vi "AutoSequencer.vi"(2 "Reinit Sequencer":bool, 7 "Auto Cluster In":T1) -> (8 "Auto Cluster Out":T1)   [LabVIEW 2020]
doc: "This VI manages the autonomous sequence. The drive base and manipulator sequencers operate in parallel. Autonomous plays are written as text files and uploaded to the roboRIO via FileZilla. The appropriate play is slected prior to the match via the FRC 4265 Dashboard. For each sequencer, each step is composed of a command and a parameter string of arbitrary length. The drive sequencer selects commands using a case structure while the subsystem sequencer selects commands using static VI references (this disparate choice is made due to conflicting memory handling and ease-of-creation tradeoffs). Error checking and handling is supported. An autonomous test mode (for simulating autonomous plays on the robot cart) is supported. Status updates are sent to the FRC Driver Station and the FRC 4265 Dashboard throughout autonomous. Note that the autonomous sequencer may be also active during the begining of TeleOperated mode, as determined by the MasterRobotModeController.vi."
uses:
  a18db1b9-ed6f-48db-83ed-89b9a31e5ef5.vi
  3b074430-bbfe-494f-99f2-72c3d74da684.vi
  a18db1b9-ed6f-48db-83ed-89b9a31e5ef5.vi/77c742ae-e671-49bb-a825-a6e8cebc9f63.vi
  3b074430-bbfe-494f-99f2-72c3d74da684.vi/77c742ae-e671-49bb-a825-a6e8cebc9f63.vi
  sensordata.vi
  driverdata.vi
  robotconstants.vi
  autonomousinfo.vi
  <vilib>/Rock Robotics/Network Tables/NT Write Value.vi
  <vilib>/Rock Robotics/Network Tables/NT Write String.vi
panel:
  in  "Type Def":T1
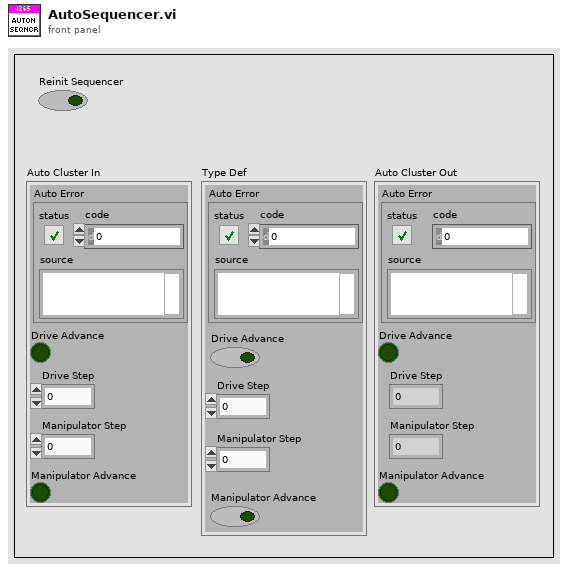
[diagram p1: front panel]
types:
  T1 = cluster{"Auto Error":errorcluster, "Drive Advance":bool, "Drive Step":i32, "Manipulator Step":i32, "Manipulator Advance":bool}
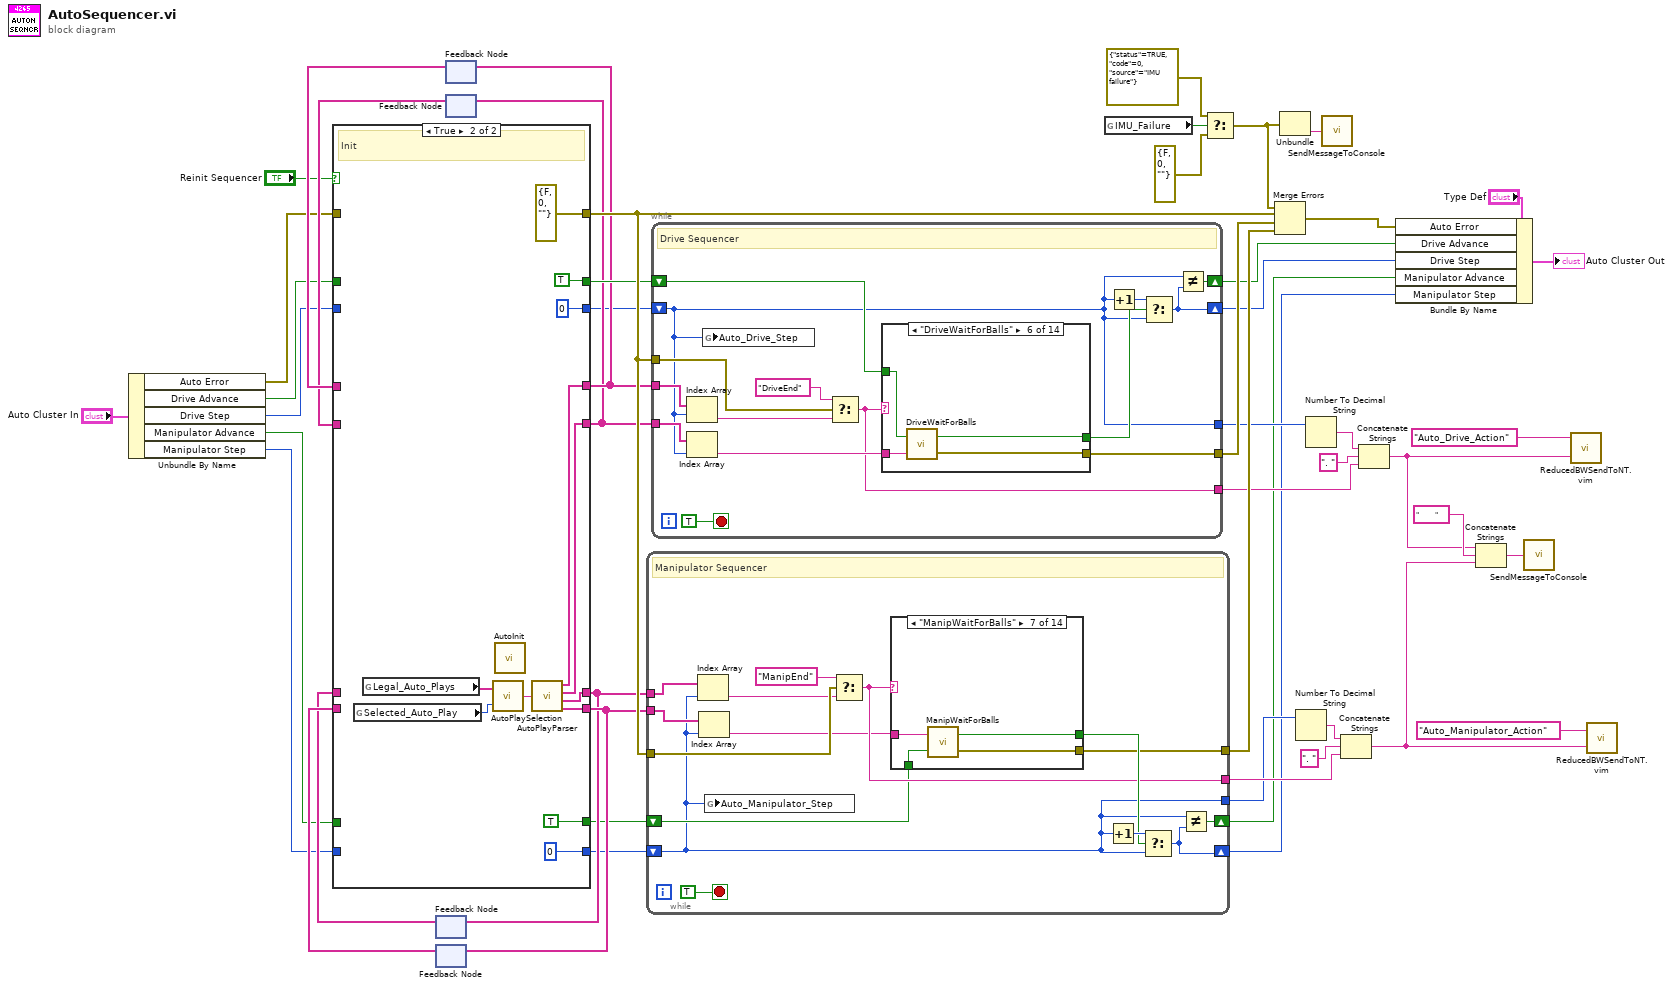
[diagram p0: block diagram]
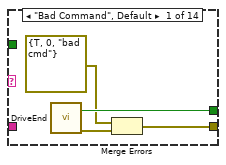
[diagram p2: hidden frame]
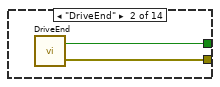
[diagram p3: hidden frame]
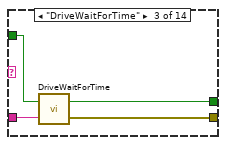
[diagram p4: hidden frame]
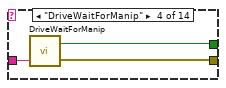
[diagram p5: hidden frame]
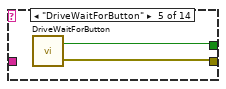
[diagram p6: hidden frame]
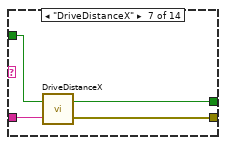
[diagram p7: hidden frame]
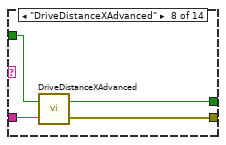
[diagram p8: hidden frame]
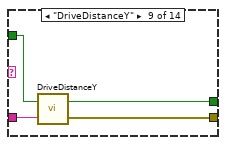
[diagram p9: hidden frame]
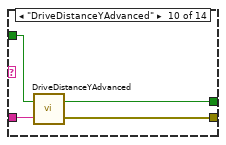
[diagram p10: hidden frame]
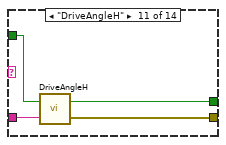
[diagram p11: hidden frame]
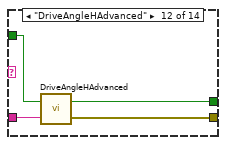
[diagram p12: hidden frame]
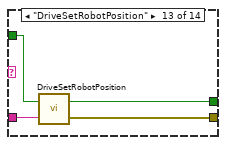
[diagram p13: hidden frame]
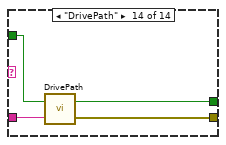
[diagram p14: hidden frame]
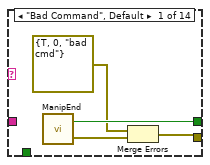
[diagram p16: hidden frame]
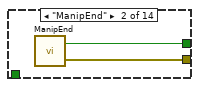
[diagram p17: hidden frame]
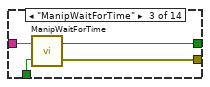
[diagram p18: hidden frame]
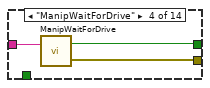
[diagram p19: hidden frame]
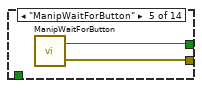
[diagram p20: hidden frame]
diagram:
  n1 = Unbundle By Name("Auto Cluster In") -> ("Auto Error"=w5:errorcluster, "Drive Advance"=w4:bool, "Drive Step"=w3:i32, "Manipulator Advance"=w2:bool, "Manipulator Step"=w1:i32)
  n2 = feedback #1() -> (w38:string[])  [unwired: 1 in]
  n3 = feedback #2() -> (w39:string[])  [unwired: 1 in]
  n4 = feedback #3() -> (w44:string[])  [unwired: 1 in]
  n5 = feedback #4() -> (w43:string[])  [unwired: 1 in]
  n6 = case shown="True" "Reinit Sequencer" {
    tunnel: w1 -> [w56 _]
    tunnel: w2 -> [w57 _]
    tunnel: [w57 TRUE ("Advance Trigger")] -> w25
    tunnel: [w56 0] -> w34
    tunnel: [w55 w63] -> w36
    tunnel: [w54 w67] -> w37
    tunnel: w38 -> [w55 _]
    tunnel: w39 -> [w54 _]
    tunnel: [w53 0] -> w40
    tunnel: w3 -> [w53 _]
    tunnel: [w52 w65] -> w41
    tunnel: [w51 w64] -> w42
    tunnel: w43 -> [w52 _]
    tunnel: w44 -> [w51 _]
    tunnel: [w50 TRUE] -> w45
    tunnel: w4 -> [w50 _]
    tunnel: [w49 errorcluster {"status"=FALSE, "code"=0, "source"=""} ("error constant")] -> w47
    tunnel: w5 -> [w49 _]
    frame False {
      # "Pass"
    }
    frame True {
      # "Init"
      n7 = global read "driverdata.vi" "Selected_Auto_Play"() -> (w61:u16)
      n8 = global read "robotconstants.vi" "Legal_Auto_Plays"() -> (w58:string[])
      n9 = call "AutoPlaySelection.vi"("Selected Auto Play"=w61, "Auto Plays"=w58) -> ("Autonomous Commands"=w60:string)
      n10 = call "AutoInit.vi"() -> ()  [unwired: 1 in]
      n11 = call "AutoPlayParser.vi"("Auto Play"=w60) -> ("Drive Command Strings"=w64:string[], "Drive Parameter Strings"=w65:string[], "Manipulator Command Strings"=w63:string[], "Manipulator Parameter Strings"=w67:string[])
    }
  }
  n12 = feedback-in #1(w36) -> ()
  n13 = feedback-in #2(w37) -> ()
  n14 = feedback-in #3(w42) -> ()
  n15 = feedback-in #4(w41) -> ()
  n16 = while {
    tunnel: w36 -> [w80]
    shift-right: [w82] -> w9
    shift-left: w34 -> [w70]
    shift-right: [w81] -> w10
    shift-left: w25 -> [w72]
    tunnel: w37 -> [w79]
    tunnel: [w74] -> w28
    tunnel: [w75] -> w48
    tunnel: w47 -> [w77]
    tunnel: [w70] -> w17
    stop <- TRUE stop-if-true
    # "Manipulator Sequencer"
    n17 = Index Array(array=w80, index=w70) -> (element=w71:string)
    n18 = Index Array(array=w79, index=w70) -> (element=w73:string)
    n19 = global write "autonomousinfo.vi" "Auto_Manipulator_Step"(w70) -> ()
    n20 = Select(t="ManipEnd", s=w77, f=w71) -> (s? t:f=w74:string)
    n21 = case shown="\"ManipWaitForBalls\"" w74 {
      tunnel: w73 -> [_ _ w94 w97 _ w103 w107 w110 w113 w116 w119 w122 w125 w128]
      tunnel: [w88 w90 w92 w96 w99 w101 w104 w109 w112 w115 w118 w121 w124 w127] -> w76
      tunnel: [w86 w89 w91 w95 w98 w100 w105 w108 w111 w114 w117 w120 w123 w126] -> w75
      tunnel: w72 -> [_ _ w93 _ _ w102 w106 _ _ _ _ _ _ _]
      frame "Bad Command", Default {
        n22 = call "ManipEnd.vi"() -> ("Error Out"=w87:errorcluster, "Advance Trigger"=w88:bool)  [unwired: 2 in]
        n23 = Merge Errors(errorcluster {"status"=TRUE, "code"=0, "source"="bad cmd"} ("Path Follow Error"), w87) -> (w86:errorcluster)
      }
      frame "ManipEnd" {
        n24 = call "ManipEnd.vi"() -> ("Error Out"=w89:errorcluster, "Advance Trigger"=w90:bool)  [unwired: 2 in]
      }
      frame "ManipWaitForTime" {
        n25 = call "ManipWaitForTime.vi"("Reinit"=w93, "Parameter String"=w94) -> ("Error Out"=w91:errorcluster, "Increment"=w92:bool)
      }
      frame "ManipWaitForDrive" {
        n26 = call "ManipWaitForDrive.vi"("Parameter String"=w97) -> ("Error Out"=w95:errorcluster, "Increment"=w96:bool)  [unwired: 1 in]
      }
      frame "ManipWaitForButton" {
        n27 = call "ManipWaitForButton.vi"() -> ("Error Out"=w98:errorcluster, "Increment"=w99:bool)  [unwired: 2 in]
      }
      frame "ManipWaitForDistance" {
        n28 = call "ManipWaitForDistance.vi"("Reinit"=w102, "Parameter String"=w103) -> ("Error Out"=w100:errorcluster, "Increment"=w101:bool)
      }
      frame "ManipWaitForBalls" {
        n29 = call "ManipWaitForBalls.vi"("Reinit"=w106, "Parameter String"=w107) -> ("Error Out"=w105:errorcluster, "Increment"=w104:bool)
      }
      frame "ManipIntake" {
        n30 = call "ManipIntake.vi"("Instruction String"=w110) -> ("Error Out"=w108:errorcluster, "Advance Trigger"=w109:bool)  [unwired: 1 in]
      }
      frame "ManipShootBalls" {
        n31 = call "ManipShootBalls.vi"("Instruction String"=w113) -> ("Error Out"=w111:errorcluster, "Advance Trigger"=w112:bool)  [unwired: 1 in]
      }
      frame "ManipForceFire" {
        n32 = call "ManipForceFire.vi"("Instruction String"=w116) -> ("Error Out"=w114:errorcluster, "Advance Trigger"=w115:bool)  [unwired: 1 in]
      }
      frame "ManipChangeState" {
        n33 = call "ManipChangeState.vi"("Instruction String"=w119) -> ("Error Out"=w117:errorcluster, "Advance Trigger"=w118:bool)  [unwired: 1 in]
      }
      frame "ManipPrespin" {
        n34 = call "ManipPrespin.vi"("Instruction String"=w122) -> ("Error Out"=w120:errorcluster, "Advance Trigger"=w121:bool)  [unwired: 1 in]
      }
      frame "ManipSetPreloadBalls" {
        n35 = call "ManipSetPreloadBalls.vi"("Parameter String"=w125) -> ("Error Out"=w123:errorcluster, "Increment"=w124:bool)  [unwired: 9 in]
      }
      frame "ManipHumanPlayerSignal" {
        n36 = call "ManipHumanPlayerSignal.vi"("Instruction String"=w128) -> ("Error Out"=w126:errorcluster, "Advance Trigger"=w127:bool)  [unwired: 9 in]
      }
    }
    n37 = Increment(x=w70) -> (x+1=w84:i32)
    n38 = Select(t=w84, s=w76, f=w70) -> (s? t:f=w82:i32)
    n39 = Not Equal?(x=w70, y=w82) -> (x != y?=w81:bool)
  }
  n40 = while {
    shift-right: [w138] -> w11
    shift-left: w40 -> [w129]
    tunnel: w42 -> [w141]
    tunnel: w41 -> [w140]
    shift-right: [w137] -> w12
    shift-left: w45 -> [w136]
    tunnel: [w130] -> w33
    tunnel: w47 -> [w134]
    tunnel: [w131] -> w46
    tunnel: [w129] -> w18
    stop <- TRUE stop-if-true
    # "Drive Sequencer"
    n41 = Index Array(array=w141, index=w129) -> (element=w133:string)
    n42 = Index Array(array=w140, index=w129) -> (element=w139:string)
    n43 = global write "autonomousinfo.vi" "Auto_Drive_Step"(w129) -> ()
    n44 = Select(t="DriveEnd", s=w134, f=w133) -> (s? t:f=w130:string)
    n45 = case shown="\"DriveWaitForBalls\"" w130 {
      tunnel: w139 -> [_ _ w151 w156 _ w162 w165 w169 w172 w177 w180 w185 w189 w193]
      tunnel: [w147 w149 w152 w154 w158 w160 w164 w168 w174 w176 w182 w184 w190 w191] -> w135
      tunnel: w136 -> [_ _ w150 _ _ w159 w166 w170 w173 w178 w181 w186 w188 w194]
      tunnel: [w145 w148 w153 w155 w157 w161 w163 w167 w171 w175 w179 w183 w187 w192] -> w131
      frame "Bad Command", Default {
        n46 = call "DriveEnd.vi"() -> ("Error Out"=w146:errorcluster, "Advance Trigger"=w147:bool)  [unwired: 2 in]
        n47 = Merge Errors(errorcluster {"status"=TRUE, "code"=0, "source"="bad cmd"} ("Path Follow Error"), w146) -> (w145:errorcluster)
      }
      frame "DriveEnd" {
        n48 = call "DriveEnd.vi"() -> ("Error Out"=w148:errorcluster, "Advance Trigger"=w149:bool)  [unwired: 2 in]
      }
      frame "DriveWaitForTime" {
        n49 = call "DriveWaitForTime.vi"("Parameter String"=w151, "Reinit"=w150) -> ("Error Out"=w153:errorcluster, "Increment"=w152:bool)
      }
      frame "DriveWaitForManip" {
        n50 = call "DriveWaitForManip.vi"("Parameter String"=w156) -> ("Error Out"=w155:errorcluster, "Increment"=w154:bool)  [unwired: 1 in]
      }
      frame "DriveWaitForButton" {
        n51 = call "DriveWaitForButton.vi"() -> ("Error Out"=w157:errorcluster, "Increment"=w158:bool)  [unwired: 2 in]
      }
      frame "DriveWaitForBalls" {
        n52 = call "DriveWaitForBalls.vi"("Parameter String"=w162, "Reinit"=w159) -> ("Error Out"=w161:errorcluster, "Increment"=w160:bool)
      }
      frame "DriveDistanceX" {
        n53 = call "DriveDistanceX.vi"("Parameter String"=w165, "Reinit"=w166) -> ("Error Out"=w163:errorcluster, "Increment"=w164:bool)
      }
      frame "DriveDistanceXAdvanced" {
        n54 = call "DriveDistanceXAdvanced.vi"("Parameter String"=w169, "Reinit"=w170) -> ("Error Out"=w167:errorcluster, "Increment"=w168:bool)
      }
      frame "DriveDistanceY" {
        n55 = call "DriveDistanceY.vi"("Parameter String"=w172, "Reinit"=w173) -> ("Error Out"=w171:errorcluster, "Increment"=w174:bool)
      }
      frame "DriveDistanceYAdvanced" {
        n56 = call "DriveDistanceYAdvanced.vi"("Parameter String"=w177, "Reinit"=w178) -> ("Error Out"=w175:errorcluster, "Increment"=w176:bool)
      }
      frame "DriveAngleH" {
        n57 = call "DriveAngleH.vi"("Parameter String"=w180, "Reinit"=w181) -> ("Error Out"=w179:errorcluster, "Increment"=w182:bool)
      }
      frame "DriveAngleHAdvanced" {
        n58 = call "DriveAngleHAdvanced.vi"("Parameter String"=w185, "Reinit"=w186) -> ("Error Out"=w183:errorcluster, "Increment"=w184:bool)
      }
      frame "DriveSetRobotPosition" {
        n59 = call "DriveSetRobotPosition.vi"("Parameter String"=w189, "Reinit"=w188) -> ("Error Out"=w187:errorcluster, "Increment"=w190:bool)
      }
      frame "DrivePath" {
        n60 = call "DrivePath.vi"("Parameter String"=w193, "Reinit"=w194) -> ("Path Follower Error"=w192:errorcluster, "Increment"=w191:bool)
      }
    }
    n61 = Increment(x=w129) -> (x+1=w142:i32)
    n62 = Select(t=w142, s=w135, f=w129) -> (s? t:f=w138:i32)
    n63 = Not Equal?(x=w129, y=w138) -> (x != y?=w137:bool)
  }
  n64 = global read "sensordata.vi" "IMU_Failure"() -> (w14:bool)
  n65 = Select(t=errorcluster {"status"=TRUE, "code"=0, "source"="IMU failure"} ("error constant"), s=w14, f=errorcluster {"status"=FALSE, "code"=0, "source"=""} ("error constant")) -> (s? t:f=w16:errorcluster)
  n66 = Merge Errors(w16, w47, w46, w48) -> (w13:errorcluster)
  n67 = Unbundle(w16) -> ("source"=w15:string)  [unwired: 2 out]
  n68 = Number To Decimal String(number=w17) -> (decimal integer string=w29:string)  [unwired: 1 in]
  n69 = Number To Decimal String(number=w18) -> (decimal integer string=w31:string)  [unwired: 1 in]
  n70 = call "SendMessageToConsole.vi"("Message String"=w15) -> ()  [unwired: 1 in]
  n71 = Concatenate Strings(w29, ". " ("string"), w28) -> (w20:string)
  n72 = Concatenate Strings(w31, ". " ("string"), w33) -> (w22:string)
  n73 = Bundle By Name(cluster="Type Def", "Auto Error"=w13, "Drive Advance"=w12, "Drive Step"=w11, "Manipulator Advance"=w10, "Manipulator Step"=w9) -> (→"Auto Cluster Out":T1)
  n74 = Concatenate Strings(w22, "        " ("string"), w20) -> (w19:string)
  n75 = call "SendMessageToConsole.vi"("Message String"=w19) -> ()  [unwired: 1 in]
  n76 = call "ReducedBWSendToNT.vim"("Value In"=w22, "NT Name"="Auto_Drive_Action" ("Name")) -> ()  [unwired: 1 out]
  n77 = call "ReducedBWSendToNT.vim"("Value In"=w20, "NT Name"="Auto_Manipulator_Action" ("Name")) -> ()  [unwired: 1 out]
